vi "write_increment_setting.vi"(8 "error in (no error)":errorcluster, 10 "increment_setting":dbl, 11 "newport_xps in":refnum<class "newport_xps.lvclass">) -> (0 "error out":errorcluster, 3 "newport_xps out":refnum<class "newport_xps.lvclass">)   [LabVIEW 2015, in "newport_xps.lvclass"]
uses:
  newport_xps.lvclass
  newport_xps.lvclass/newport_xps.ctl
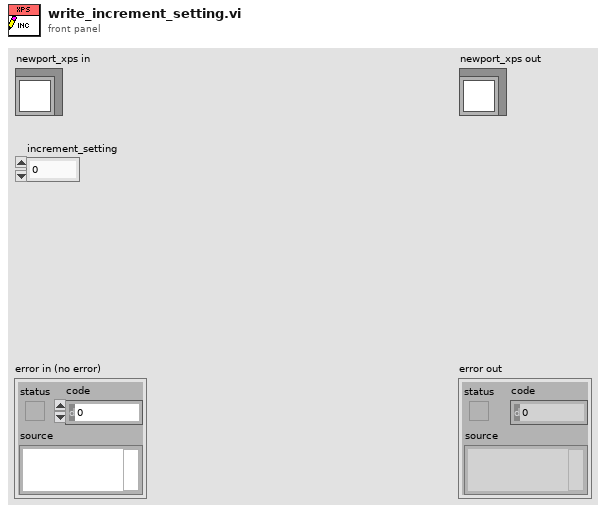
[diagram p1: front panel]
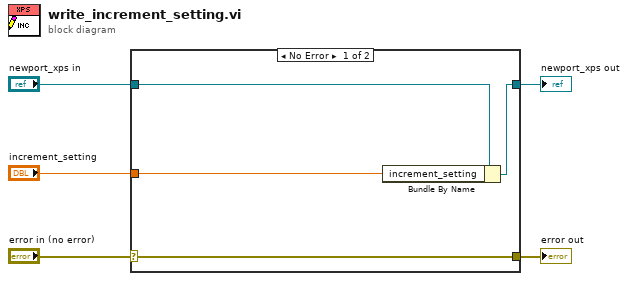
[diagram p0: block diagram]
diagram:
  n1 = case shown="No Error" "error in (no error)" {
    selector: "error in (no error)" -> [w9 w10]
    tunnel: [w9 w10] -> w4
    tunnel: [w7 w11] -> w2
    tunnel: "newport_xps in" -> [w8 w11]
    tunnel: "increment_setting" -> [w6 _]
    frame No Error {
      n2 = Bundle By Name(cluster=w8, "increment_setting"=w6) -> (w7:refnum<class "newport_xps.lvclass">)
    }
    frame Error {
    }
  }
  "error out" <- w4
  "newport_xps out" <- w2
